vi "PYTHON Get Variables__ogtk.vi"(4 "error in (no error)":errorcluster, 7 "Python Session in":T1) -> (0 "error out":errorcluster, 1 "types":string[](array[string]), 2 "names":string[](array[string]), 3 "Python Session out":T1)   [LabVIEW 2014]
doc: "This function retrieves a list of all currently defined local variables and their type. Locale variables can have been set previously with the PYTHON Set <type> Data.vi functions and/or been generated or updated by a previous call to PYTHON Execute Script.vi."
uses:
  <userlib>/_OpenG.lib/labpython/labpython.llb/PYTHON Session Refnum__ogtk.ctl
  <userlib>/_OpenG.lib/labpython/lvpython.dll
panel:
  # "PYTHON Get Variables.vi\n\nRetrieves the variable names and types from the session context\n\nCopyright (C) 2002 Rolf Kalbermatter rolf.kalbermatter@citeng.com\nCopyright (C) 2002 James Kring jim@jimkring.com\n\nPlease visit http://www.OpenG.org to learn about the\nOpen Source LabVIEW software movement.\n\nThis library is free software; you can redistribute it and/or\nmodify it under the terms of the GNU Lesser General Public\nLicense as published by the Free Software Foundation; either\nversion 2.1 of the License, or (at your option) any later version.\nThis library is distributed in the hope that it will be useful,\nbut WITHOUT ANY WARRANTY; without even the implied warranty of\nMERCHANTABILITY or FITNESS FOR A PARTICULAR PURPOSE. See the GNU\nLesser General Public License for more details.\nYou should have received a copy of the GNU Lesser General Public\nLicense along with this library; if not, write to the Free Software\nFoundation, Inc., 59 Temple Place, Suite 330, Boston, MA 02111-1307 USA"
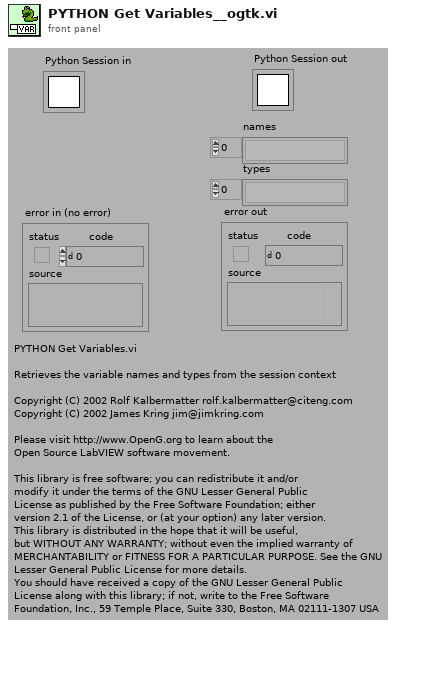
[diagram p1: front panel]
types:
  T1 = typedef "PYTHON Session Refnum__ogtk.ctl" = refnum<k1>
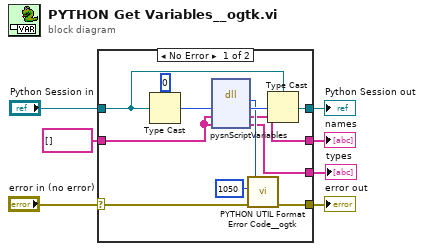
[diagram p0: block diagram]
diagram:
  n1 = case shown="No Error" "error in (no error)" {
    selector: "error in (no error)" -> [w18 w22]
    tunnel: [w12 w21] -> w4
    tunnel: [w16 w22] -> w6
    tunnel: "Python Session in" -> [w11 w21]
    tunnel: string[] [] ("names") -> [w8 w20]
    tunnel: [w10 w20] -> w2
    tunnel: [w9 w20] -> w1
    frame No Error {
      n2 = Type Cast(type=u32 0 ("session"), x=w11) -> (*(type *) &x=w13:u32)
      n3 = dll-call lib="C:/Program Files (x86)/National Instruments/LabVIEW 2014/user.lib/_OpenG.lib/labpython/lvpython.*" fn="pysnScriptVariables"("session"=w13, "names"=w8, "names"=w8) -> (w17:i32, "session"=w19:u32, "names"=w10:string[], "names"=w9:string[])  [unwired: 3 in, 2 out]
      n4 = call <userlib>:"PYTHON UTIL Format Error Code__ogtk.vi"("error in (no error)"=w18, "code"=1050, "Bool32"=w17) -> ("error out"=w16:errorcluster)  [unwired: 4 in]
      n5 = Type Cast(type=w11, x=w19) -> (*(type *) &x=w12:T1)
    }
    frame Error {
    }
  }
  "error out" <- w6
  "Python Session out" <- w4
  "names" <- w2
  "types" <- w1
